vi "DAQ.Write AO.vi"(8 "error in (no error)":errorcluster, 10 "AO []":waveform(dbl)[](array[waveform]), 11 "Instrument.DAQ in":refnum<class "Instrument.DAQ.lvclass">) -> (0 "error out":errorcluster, 2 "AO out []":waveform(dbl)[](array[waveform]), 3 "Instrument.DAQ out":refnum<class "Instrument.DAQ.lvclass">, 4 "AO time (ms)":u32=53)   [LabVIEW 2019, in "Instrument.Lockin.lvlib" / "Instrument.DAQ.lvclass"]
uses:
  Instrument.DAQ.lvclass
  Instrument.DAQ.lvclass/Instrument.DAQ.ctl
  <vilib>/DAQmx/write.llb/DAQmx Write (Analog 1D Wfm NChan NSamp).vi
  <vilib>/Waveform/WDTOps.llb/WDT Append Waveforms DBL.vi
  <vilib>/DAQmx/miscellaneous.llb/DAQmx Fill In Error Info.vi
panel:
  out "AO (previous)":waveform(dbl)[](array[waveform])
  out "Waveform Graph":waveform(dbl)[](graph)
  out "P Check":bool[](array[boolean])
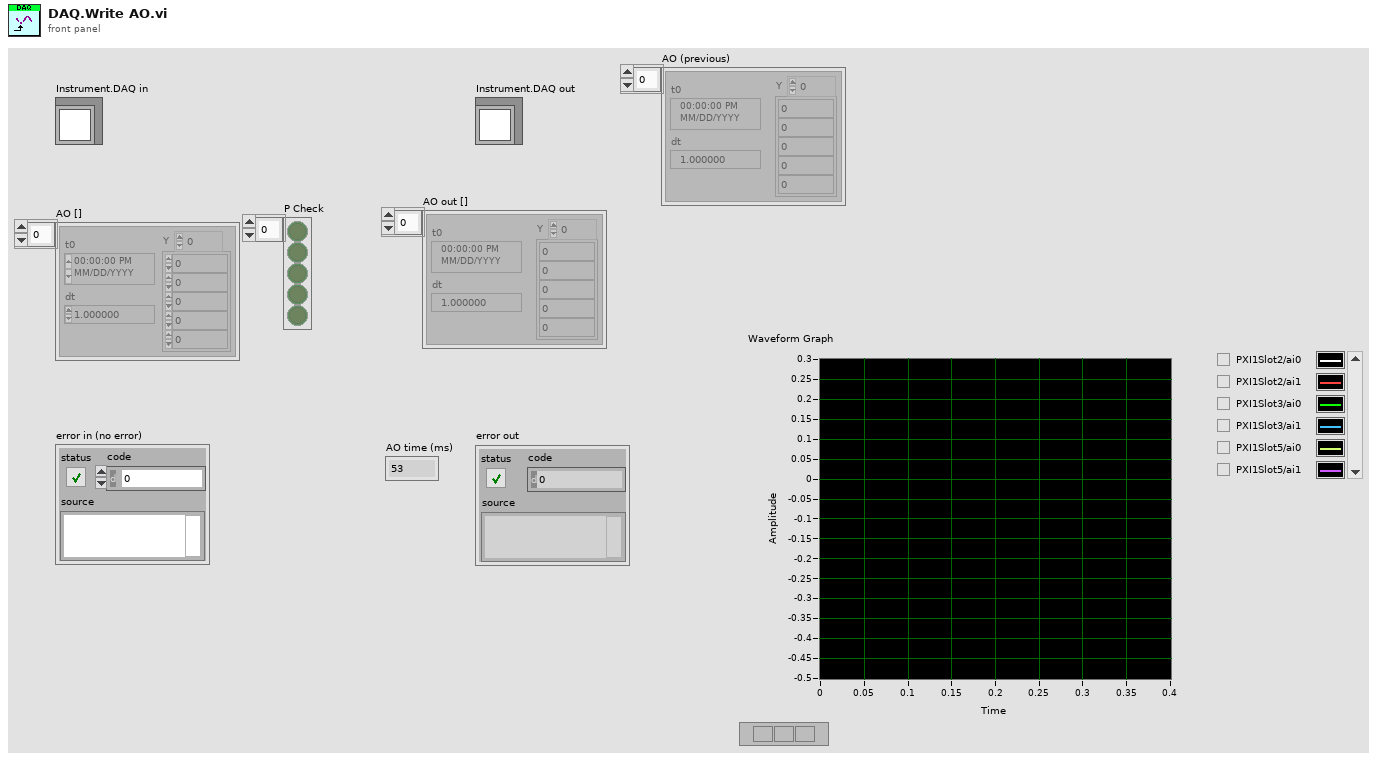
[diagram p1: front panel]
types:
  T1 = enum16{"static", "dynamic", "dynamic asynchronous"}
  T2 = typedef "Instrument.Lockin.lvlib/Instrument.DAQ.lvclass/DAQ.Type--enum.ctl" = enum16{"None", "USB-4431", "PXI-446x"}
  T3 = typedef "Instrument.Lockin.lvlib/Instrument.DAQ.lvclass/AO.Channel--Cluster--Array.ctl" = T4[]
  T4 = typedef "Instrument.Lockin.lvlib/Instrument.DAQ.lvclass/AO.Channel--Cluster.ctl" = cluster{"Enable?":bool, "Channel":i32, "Amplitude":dbl, "Offset":dbl, "Frequency":dbl, "Phase":dbl, "Function":T5, "Sweeping?":bool}
  T5 = typedef "Instrument.Lockin.lvlib/Instrument.DAQ.lvclass/AO.Channel.Function--Enum.ctl" = enum16{"Sine", "Triangle", "Square"}
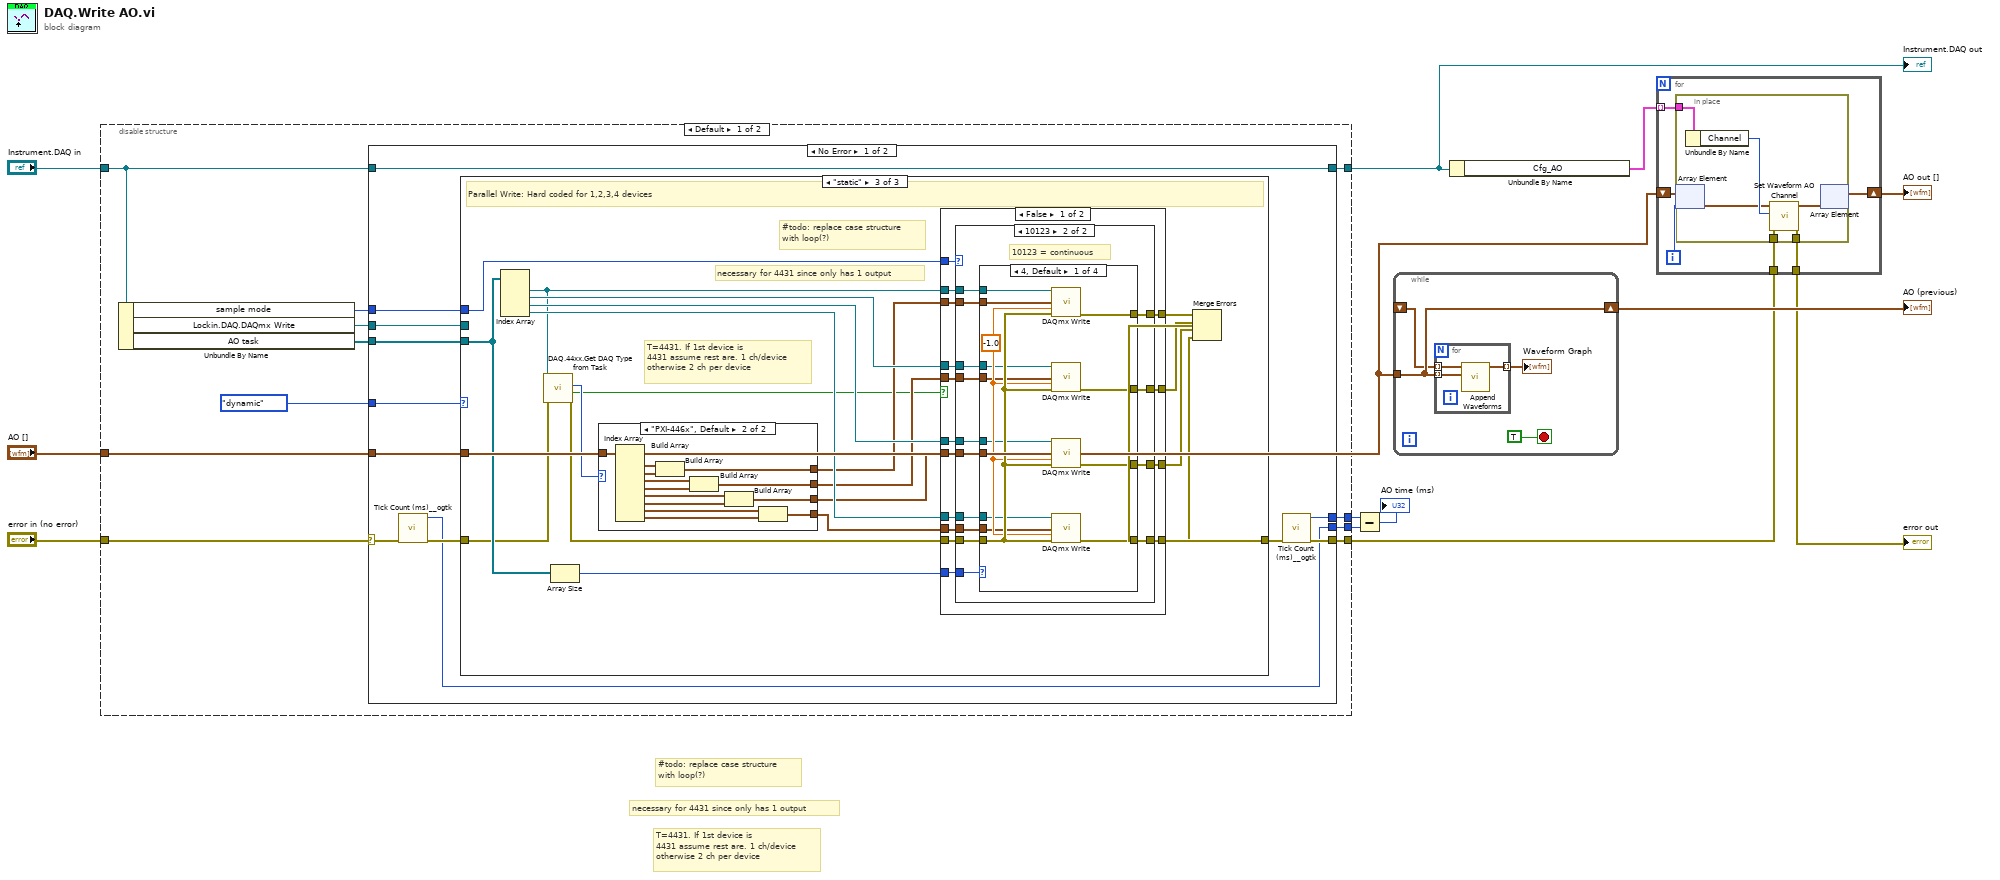
[diagram p0: block diagram]
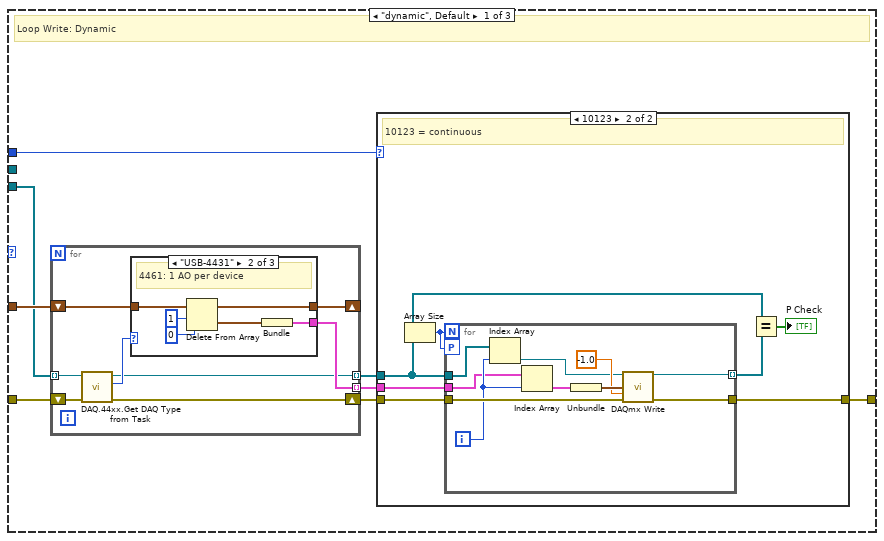
[diagram p2: hidden frame]
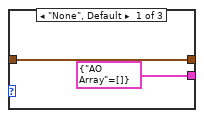
[diagram p3: hidden frame]
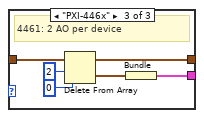
[diagram p4: hidden frame]
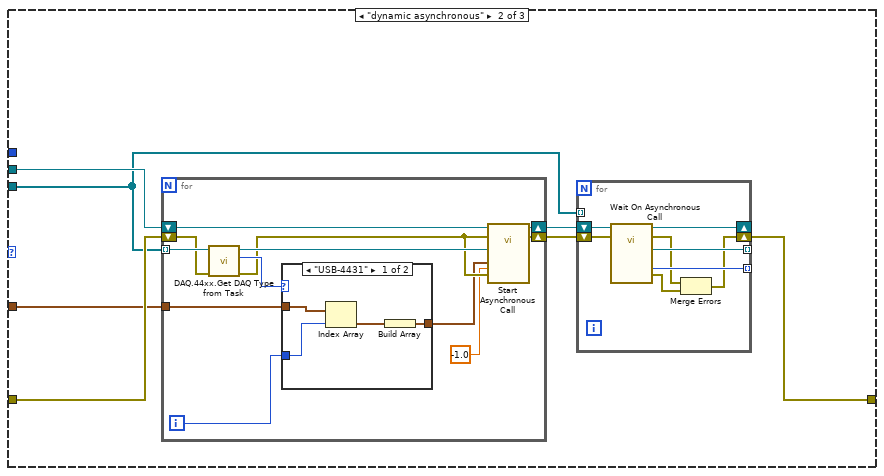
[diagram p6: hidden frame]
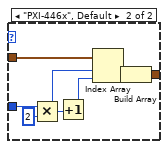
[diagram p7: hidden frame]
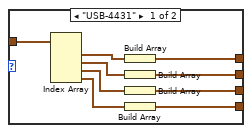
[diagram p8: hidden frame]
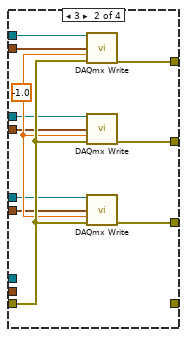
[diagram p10: hidden frame]
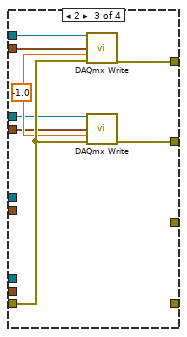
[diagram p11: hidden frame]
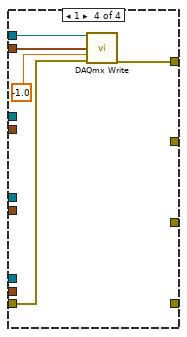
[diagram p12: hidden frame]
diagram:
  # "#todo: replace case structure\nwith loop(?)"
  # "T=4431. If 1st device is \n4431 assume rest are. 1 ch/device\notherwise 2 ch per device"
  # "necessary for 4431 since only has 1 output"
  n1 = disable-structure shown="Default" {
    disable-tunnel: [w23 w238] -> w2
    disable-tunnel: "Instrument.DAQ in" -> [w21 w237]
    disable-tunnel: "AO []" -> [w22 _]
    disable-tunnel: "error in (no error)" -> [w16 w238]
    disable-tunnel: [w20 w237] -> w6
    disable-tunnel: [w19 _] -> w12
    disable-tunnel: [w18 _] -> w9
    frame condition #0 (active) {
      n2 = Unbundle By Name(w21) -> ("sample mode"=w13:i32, "Lockin.DAQ.DAQmx Write"=w15:refnum<vi>, "AO task"=w17:refnum<k21>[])
      n3 = case shown="No Error" w16 {
        selector: w16 -> [w29 w235]
        tunnel: [w32 w235] -> w23
        tunnel: w22 -> [w34 _]
        tunnel: w17 -> [w35 _]
        tunnel: w21 -> [w30 w236]
        tunnel: [w30 w236] -> w20
        tunnel: [w31 _] -> w19
        tunnel: [w26 _] -> w18
        tunnel: w15 -> [w27 _]
        tunnel: T1."dynamic" ("Enum") -> [w25 _]
        tunnel: w13 -> [w24 _]
        frame No Error {
          n4 = call <userlib>:"Tick Count (ms)__ogtk.vi"("error in (no error)"=w29) -> ("error out"=w28:errorcluster, "millisecond timer value"=w26:u32)  [unwired: 9 in]
          n5 = case shown="\"static\"" w25 {
            tunnel: w35 -> [w37 w84 w143]
            tunnel: w34 -> [w41 w86 w142]
            tunnel: [w40 w85 w141] -> w33
            tunnel: w28 -> [w43 w88 w126]
            tunnel: w27 -> [_ w87 _]
            tunnel: w24 -> [w36 _ w123]
            frame "dynamic", Default {
              # "Loop Write: Dynamic"
              n6 = for {
                tunnel: [w47] -> w39 mode=indexing
                shift-right: [w50] -> w42
                shift-left: w43 -> [w51]
                tunnel: w37 -> [w46] mode=indexing
                shift-right: [w45] -> _
                shift-left: w41 -> [w49]
                tunnel: [w44] -> w38 mode=indexing
                n7 = call "DAQ.44xx.Get DAQ Type from Task.vi"("error in (no error)"=w51, "Task in"=w46) -> ("error out"=w50:errorcluster, "DAQ Type"=w48:T2, "Task out"=w44:refnum<k21>)  [unwired: 6 in, 1 out]
                n8 = case shown="\"USB-4431\"" w48 {
                  tunnel: w49 -> [w53 w59 w65]
                  tunnel: [w53 w58 w64] -> w45
                  tunnel: [cluster{"AO Array":waveform(dbl)[]} {"AO Array"=[]} w56 w61] -> w47
                  frame "None", Default {
                  }
                  frame "USB-4431" {
                    # "4461: 1 AO per device"
                    n9 = Delete From Array(array=w59, length=1, index=0) -> (deleted portion=w55:waveform(dbl)[], array with subset deleted=w58:waveform(dbl)[])
                    n10 = Bundle("AO []"=w55) -> (w56:cluster{"AO []":waveform(dbl)[]})  [unwired: 1 in]
                  }
                  frame "PXI-446x" {
                    # "4461: 2 AO per device"
                    n11 = Delete From Array(array=w65, length=2, index=0) -> (deleted portion=w62:waveform(dbl)[], array with subset deleted=w64:waveform(dbl)[])
                    n12 = Bundle("AO []"=w62) -> (w61:cluster{"AO []":waveform(dbl)[]})  [unwired: 1 in]
                  }
                }
              }
              n13 = case shown="10123" w36 {
                tunnel: [w66 w71] -> w40
                tunnel: w38 -> [_ w70]
                tunnel: w39 -> [_ w73]
                tunnel: w42 -> [w66 w72]
                frame 10178, Default {
                  # "10178 = finite sample mode (IV\nmode). Do not try to write\nmore samples to the buffer"
                }
                frame 10123 {
                  # "10123 = continuous"
                  n14 = Array Size(array=w70) -> (size(s)=w68:i32)
                  n15 = for {
                    N: w68 -> [_]
                    tunnel: w70 -> [w76]
                    tunnel: w73 -> [w77]
                    tunnel: w72 -> [w83]
                    tunnel: [w74] -> w71
                    workers-P: w68 -> [_]
                    tunnel: [w75] -> w67 mode=indexing
                    i -> [w78]
                    n16 = Index Array(array=w76, index=w78) -> (element=w79:refnum<k21>)
                    n17 = Index Array(array=w77, index=w78) -> (element=w80:cluster{"AO []":waveform(dbl)[]})
                    n18 = Unbundle(w80) -> ("AO []"=w82:waveform(dbl)[])
                    n19 = call-poly <vilib>:"DAQmx Write.vi"("task/channels in"=w79, "data"=w82, "timeout"=-1.0, "error in"=w83) -> ("task out"=w75:refnum<k21>, "error out"=w74:errorcluster)  [unwired: 9 in, 1 out]
                  }
                  n20 = Equal?(x=w70, y=w67) -> (x = y?=→"P Check":bool[])
                }
              }
            }
            frame "dynamic asynchronous" {
              n21 = for {
                shift-right: [w102] -> w89
                shift-left: w88 -> [w96]
                shift-right: [w101] -> w90
                shift-left: w87 -> [w100]
                tunnel: w84 -> [w98] mode=indexing
                tunnel: w86 -> [w94]
                i -> [w93]
                n22 = call "DAQ.44xx.Get DAQ Type from Task.vi"("error in (no error)"=w96, "Task in"=w98) -> ("error out"=w95:errorcluster, "DAQ Type"=w99:T2, "Task out"=w97:refnum<k21>)  [unwired: 6 in, 1 out]
                n23 = case shown="\"USB-4431\"" w99 {
                  tunnel: [w105 w112] -> w92
                  tunnel: w94 -> [w104 w111]
                  tunnel: w93 -> [w103 w109]
                  frame "USB-4431" {
                    n24 = Index Array(array=w104, index=w103) -> (element=w106:waveform(dbl))
                    n25 = Build Array(w106) -> (w105:waveform(dbl)[])
                  }
                  frame "PXI-446x", Default {
                    n26 = Multiply(x=w109, y=2) -> (x*y=w108:i32)
                    n27 = Increment(x=w108) -> (x+1=w107:i32)
                    n28 = Index Array(array=w111, index #1=w108, index #2=w107) -> (element #1=w113:waveform(dbl), element #2=w114:waveform(dbl))
                    n29 = Build Array(w113, w114) -> (w112:waveform(dbl)[])
                  }
                }
                n30 = call-by-ref "Start Asynchronous Call"(reference=w100, error in=w95, "Refnum in"=w97, "data"=w92, "timeout"=-1.0, 11:"error in (no error)"=w95) -> (reference out=w101:refnum<vi>, error out=w102:errorcluster)  [unwired: 8 in, 4 out]
              }
              n31 = for {
                shift-right: [w115] -> w85
                shift-left: w89 -> [w121]
                shift-right: [w120] -> _
                shift-left: w90 -> [w122]
                tunnel: [w119] -> _ mode=indexing
                tunnel: [w118] -> _ mode=indexing
                tunnel: w84 -> [_] mode=indexing
                n32 = call-by-ref "Wait On Asynchronous Call"(reference=w122, error in=w121) -> (reference out=w120:refnum<vi>, error out=w116:errorcluster, "Refnum out"=w119:refnum<k21>, "number of samples written per channel"=w118:u32, 15:"error out"=w117:errorcluster)  [unwired: 12 in, 1 out]
                n33 = Merge Errors(w116, w117) -> (w115:errorcluster)
              }
            }
            frame "static" {
              # "#todo: replace case structure\nwith loop(?)"
              # "T=4431. If 1st device is \n4431 assume rest are. 1 ch/device\notherwise 2 ch per device"
              # "necessary for 4431 since only has 1 output"
              # "Parallel Write: Hard coded for 1,2,3,4 devices"
              n34 = Index Array(array=w143) -> (element #1=w136:refnum<k21>, element #2=w140:refnum<k21>, element #3=w139:refnum<k21>, element #4=w138:refnum<k21>)  [unwired: 4 in]
              n35 = call "DAQ.44xx.Get DAQ Type from Task.vi"("error in (no error)"=w126, "Task in"=w136) -> ("error out"=w125:errorcluster, "DevIsSimulated"=w127:bool, "DAQ Type"=w132:T2)  [unwired: 6 in, 1 out]
              n36 = Array Size(array=w143) -> (size(s)=w137:i32)
              n37 = case shown="\"PXI-446x\", Default" w132 {
                tunnel: [w152 w158] -> w134
                tunnel: [w151 w157] -> w135
                tunnel: [w150 w156] -> w124
                tunnel: [w148 w154] -> w133
                tunnel: w142 -> [w147 w153]
                frame "USB-4431" {
                  n38 = Index Array(array=w147) -> (element #1=w149:waveform(dbl), element #2=w146:waveform(dbl), element #3=w145:waveform(dbl), element #4=w144:waveform(dbl))  [unwired: 4 in]
                  n39 = Build Array(w149) -> (w148:waveform(dbl)[])
                  n40 = Build Array(w146) -> (w152:waveform(dbl)[])
                  n41 = Build Array(w145) -> (w151:waveform(dbl)[])
                  n42 = Build Array(w144) -> (w150:waveform(dbl)[])
                }
                frame "PXI-446x", Default {
                  n43 = Index Array(array=w153) -> (element #1=w155:waveform(dbl), element #2=w165:waveform(dbl), element #3=w164:waveform(dbl), element #4=w163:waveform(dbl), element #5=w162:waveform(dbl), element #6=w161:waveform(dbl), element #7=w160:waveform(dbl), element #8=w159:waveform(dbl))  [unwired: 8 in]
                  n44 = Build Array(w155, w165) -> (w154:waveform(dbl)[])
                  n45 = Build Array(w164, w163) -> (w158:waveform(dbl)[])
                  n46 = Build Array(w162, w161) -> (w157:waveform(dbl)[])
                  n47 = Build Array(w160, w159) -> (w156:waveform(dbl)[])
                }
              }
              n48 = case shown="False" w127 {
                tunnel: w140 -> [w180 _]
                tunnel: w139 -> [w179 _]
                tunnel: w138 -> [w178 _]
                tunnel: w137 -> [w177 _]
                tunnel: w136 -> [w176 _]
                tunnel: w124 -> [w175 _]
                tunnel: w135 -> [w174 _]
                tunnel: w134 -> [w173 _]
                tunnel: w133 -> [w172 _]
                tunnel: w125 -> [w171 w234]
                tunnel: [w170 _] -> w131
                tunnel: [w169 _] -> w130
                tunnel: [w168 w234] -> w129
                tunnel: [w166 _] -> w128
                tunnel: w123 -> [w167 _]
                frame False {
                  n49 = case shown="10123" w167 {
                    tunnel: w180 -> [_ w195]
                    tunnel: w179 -> [_ w194]
                    tunnel: w178 -> [_ w193]
                    tunnel: [w181 w192] -> w168
                    tunnel: [_ w191] -> w169
                    tunnel: [_ w190] -> w170
                    tunnel: [_ w189] -> w166
                    tunnel: w177 -> [_ w188]
                    tunnel: w176 -> [_ w187]
                    tunnel: w175 -> [_ w186]
                    tunnel: w174 -> [_ w185]
                    tunnel: w173 -> [_ w184]
                    tunnel: w172 -> [_ w183]
                    tunnel: w171 -> [w181 w182]
                    frame 10178, Default {
                      # "10178 = finite sample mode (IV\nmode). Do not try to write\nmore samples to the buffer"
                    }
                    frame 10123 {
                      # "10123 = continuous"
                      n50 = case shown="4, Default" w188 {
                        tunnel: w182 -> [w209 w220 w228 w233]
                        tunnel: w195 -> [w207 w218 w226 _]
                        tunnel: w194 -> [w206 w217 _ _]
                        tunnel: w193 -> [w205 _ _ _]
                        tunnel: w184 -> [w204 w216 w225 _]
                        tunnel: w185 -> [w203 w215 _ _]
                        tunnel: w186 -> [w202 _ _ _]
                        tunnel: [w201 w214 w224 w231] -> w192
                        tunnel: [w200 w213 w223 _] -> w191
                        tunnel: [w199 w212 _ _] -> w190
                        tunnel: [w198 _ _ _] -> w189
                        tunnel: w187 -> [w197 w211 w222 w230]
                        tunnel: w183 -> [w196 w210 w221 w229]
                        frame 4, Default {
                          w208 = -1.0 ("timeout")
                          n51 = call-poly <vilib>:"DAQmx Write.vi"("task/channels in"=w197, "data"=w196, "timeout"=w208, "error in"=w209) -> ("error out"=w201:errorcluster)  [unwired: 9 in, 2 out]
                          n52 = call-poly <vilib>:"DAQmx Write.vi"("task/channels in"=w207, "data"=w204, "timeout"=w208, "error in"=w209) -> ("error out"=w200:errorcluster)  [unwired: 9 in, 2 out]
                          n53 = call-poly <vilib>:"DAQmx Write.vi"("task/channels in"=w206, "data"=w203, "timeout"=w208, "error in"=w209) -> ("error out"=w199:errorcluster)  [unwired: 9 in, 2 out]
                          n54 = call-poly <vilib>:"DAQmx Write.vi"("task/channels in"=w205, "data"=w202, "timeout"=w208, "error in"=w209) -> ("error out"=w198:errorcluster)  [unwired: 9 in, 2 out]
                        }
                        frame 3 {
                          w219 = -1.0 ("timeout")
                          n55 = call-poly <vilib>:"DAQmx Write.vi"("task/channels in"=w211, "data"=w210, "timeout"=w219, "error in"=w220) -> ("error out"=w214:errorcluster)  [unwired: 9 in, 2 out]
                          n56 = call-poly <vilib>:"DAQmx Write.vi"("task/channels in"=w218, "data"=w216, "timeout"=w219, "error in"=w220) -> ("error out"=w213:errorcluster)  [unwired: 9 in, 2 out]
                          n57 = call-poly <vilib>:"DAQmx Write.vi"("task/channels in"=w217, "data"=w215, "timeout"=w219, "error in"=w220) -> ("error out"=w212:errorcluster)  [unwired: 9 in, 2 out]
                        }
                        frame 2 {
                          w227 = -1.0 ("timeout")
                          n58 = call-poly <vilib>:"DAQmx Write.vi"("task/channels in"=w222, "data"=w221, "timeout"=w227, "error in"=w228) -> ("error out"=w224:errorcluster)  [unwired: 9 in, 2 out]
                          n59 = call-poly <vilib>:"DAQmx Write.vi"("task/channels in"=w226, "data"=w225, "timeout"=w227, "error in"=w228) -> ("error out"=w223:errorcluster)  [unwired: 9 in, 2 out]
                        }
                        frame 1 {
                          n60 = call-poly <vilib>:"DAQmx Write.vi"("task/channels in"=w230, "data"=w229, "timeout"=-1.0, "error in"=w233) -> ("error out"=w231:errorcluster)  [unwired: 9 in, 2 out]
                        }
                      }
                    }
                  }
                }
                frame True {
                }
              }
              n61 = Merge Errors(w129, w130, w131, w128) -> (w141:errorcluster)
            }
          }
          n62 = call <userlib>:"Tick Count (ms)__ogtk.vi"("error in (no error)"=w33) -> ("error out"=w32:errorcluster, "millisecond timer value"=w31:u32)  [unwired: 9 in]
        }
        frame Error {
        }
      }
    }
    frame condition #1 {
    }
  }
  "Instrument.DAQ out" <- w6
  n63 = Subtract(x=w12, y=w9) -> (x-y=→"AO time (ms)":u32)
  n64 = while {
    shift-right: [w240] -> w7
    shift-left: _ -> [w239]
    tunnel: "AO []" -> [w240]
    stop <- TRUE stop-if-true
    n65 = for {
      tunnel: [w245] -> w241 mode=indexing
      tunnel: w239 -> [w244] mode=indexing
      tunnel: w240 -> [w243] mode=indexing
      n66 = call-poly <vilib>:"Append Waveforms.vi"("waveform B"=w243, "waveform A"=w244) -> ("waveform out"=w245:waveform(dbl))  [unwired: 8 in, 1 out]
    }
    "Waveform Graph" <- w241
  }
  "AO (previous)" <- w7
  n67 = Unbundle By Name(w6) -> ("Cfg_AO"=w5:T3)
  n68 = for {
    tunnel: w5 -> [w251] mode=indexing
    tunnel: w2 -> [w248]
    tunnel: [w247] -> w1
    shift-right: [w246] -> w3
    shift-left: "AO []" -> [w249]
    i -> [w250]
    n69 = in-place {
      in-place-border: w251 -> [w257]
      in-place-border: w248 -> [w253]
      in-place-border: [w252] -> w247
      n70 = in-place-array #1(w249, w250) -> (w255:waveform(dbl))
      n71 = Unbundle By Name(w257) -> ("Channel"=w256:i32)
      n72 = call "Set Waveform AO Channel.vi"("error in (no error)"=w253, "AO Channel"=w256, "Waveform in"=w255) -> ("error out"=w252:errorcluster, "Waveform out"=w254:waveform(dbl))  [unwired: 7 in]
      n73 = in-place-array #1(w254) -> (w246:waveform(dbl)[])  [unwired: 1 out]
    }
  }
  "error out" <- w1
  "AO out []" <- w3
